vi "Get Model Info - from DLL.vi"(0 "Model Filepath":path, 4 "Models":string[](array[string]), 5 "Error (in)":errorcluster) -> (14 "DLL Inports":string[](array[string]), 15 "DLL Outports":string[](array[string]), 16 "DLL Parameters":string[](array[string]), 17 "DLL Signals":string[](array[string]), 19 "Error (out)":errorcluster)   [LabVIEW 2016, in "System Mapping Tool.lvlib"]
uses:
  System Mapping Tool.lvlib
  <vilib>/Model Interface Toolkit/Get Inport Paths.vi
  <vilib>/Model Interface Toolkit/Get Outport Paths.vi
  <vilib>/Model Interface Toolkit/Get Parameter Paths.vi
  <vilib>/Model Interface Toolkit/Get Signal Paths.vi
  <vilib>/Model Interface Toolkit/Model Interface Toolkit.lvclass
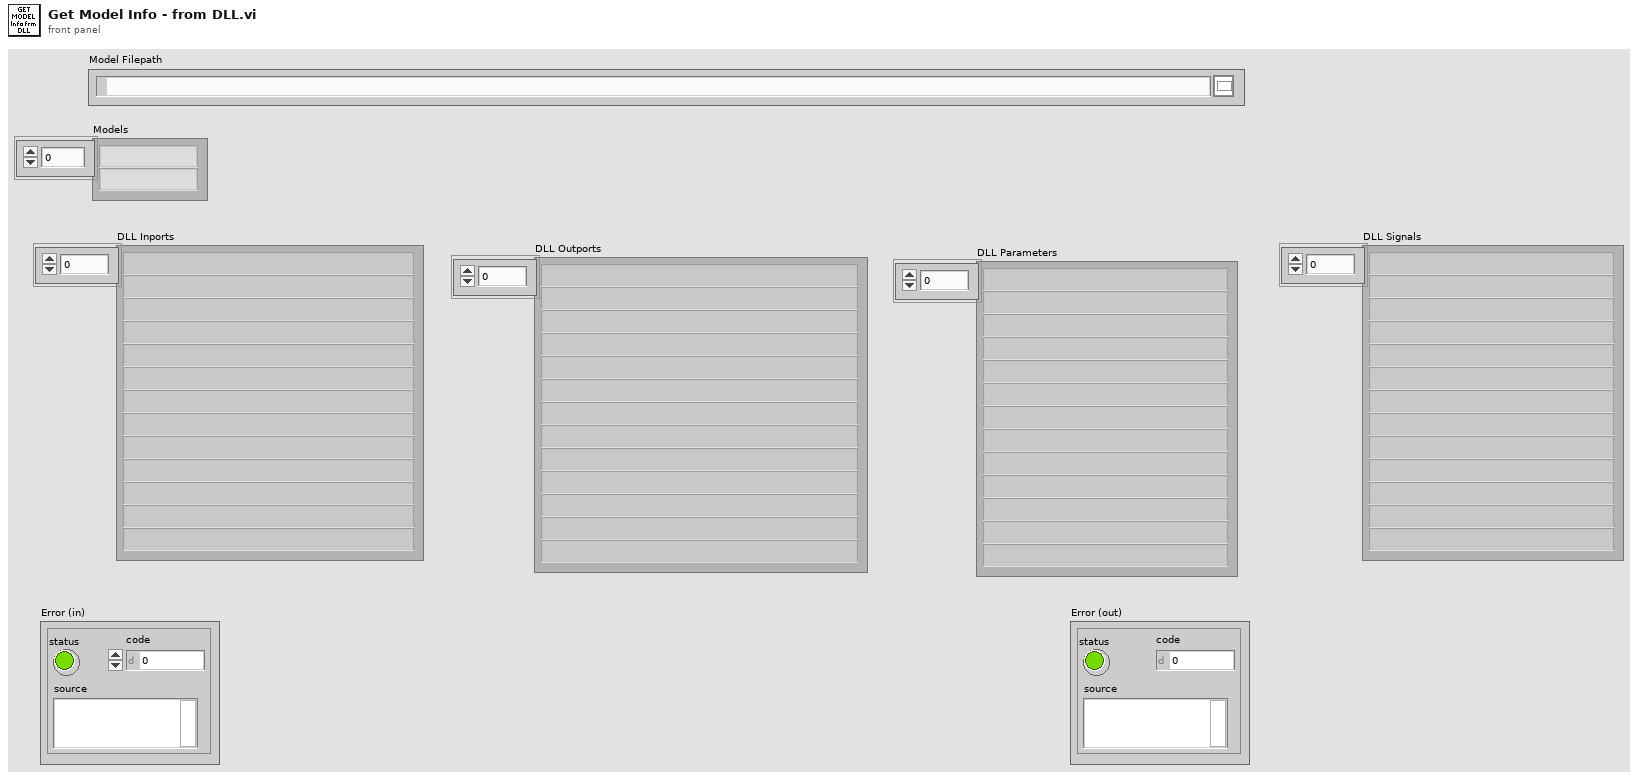
[diagram p1: front panel]
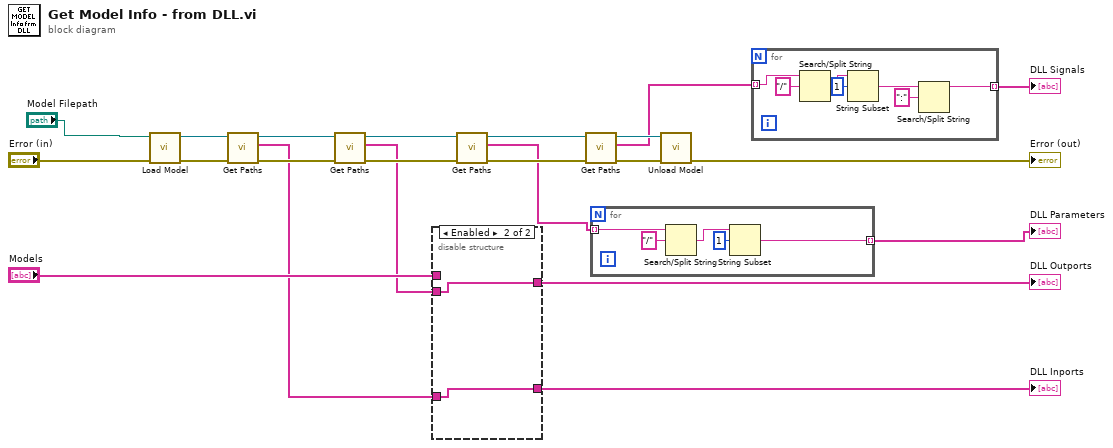
[diagram p0: block diagram]
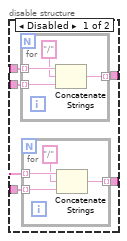
[diagram p2: hidden frame]
diagram:
  n1 = call <vilib>:"Load Model.vi"("error in (no error)"="Error (in)", "Model Path"="Model Filepath") -> ("error out"=w13:errorcluster, "Model out"=w14:refnum<class "Model Interface Toolkit.lvclass">)  [unwired: 8 in]
  n2 = call-poly <vilib>:"Get Paths.vi"("error in (no error)"=w13, "Model in"=w14) -> ("error out"=w12:errorcluster, "Inport Paths"=w9:string[], "Model out"=w15:refnum<class "Model Interface Toolkit.lvclass">)  [unwired: 7 in]
  n3 = call-poly <vilib>:"Get Paths.vi"("error in (no error)"=w12, "Model in"=w15) -> ("error out"=w11:errorcluster, "Outport Paths"=w10:string[], "Model out"=w16:refnum<class "Model Interface Toolkit.lvclass">)  [unwired: 7 in]
  n4 = disable-structure shown="Enabled" {
    disable-tunnel: w10 -> [w27 w37]
    disable-tunnel: [w26 w37] -> w20
    disable-tunnel: w9 -> [w25 w36]
    disable-tunnel: [w24 w36] -> w19
    disable-tunnel: "Models" -> [w23 _]
    frame Disabled {
      n5 = for {
        tunnel: w23 -> [w35] mode=indexing
        tunnel: w27 -> [w34] mode=indexing
        tunnel: [w32] -> w26 mode=indexing
        n6 = Concatenate Strings(w35, "/" ("string"), w34) -> (w32:string)
      }
      n7 = for {
        tunnel: w23 -> [w31] mode=indexing
        tunnel: w25 -> [w30] mode=indexing
        tunnel: [w28] -> w24 mode=indexing
        n8 = Concatenate Strings(w31, "/" ("string"), w30) -> (w28:string)
      }
    }
    frame Enabled {
    }
  }
  "DLL Inports" <- w19
  "DLL Outports" <- w20
  n9 = call-poly <vilib>:"Get Paths.vi"("error in"=w11, "Model in"=w16) -> ("error out"=w8:errorcluster, "Parameter Paths"=w4:string[], "Model out"=w6:refnum<class "Model Interface Toolkit.lvclass">)  [unwired: 7 in]
  n10 = call-poly <vilib>:"Get Paths.vi"("error in"=w8, "Model in"=w6) -> ("error out"=w7:errorcluster, "Signal Paths"=w2:string[], "Model out"=w5:refnum<class "Model Interface Toolkit.lvclass">)  [unwired: 7 in]
  n11 = for {
    tunnel: w4 -> [w42] mode=indexing
    tunnel: [w39] -> w3 mode=indexing
    n12 = Search/Split String(string=w42, search string/char (-)="/") -> (match + rest of string=w38:string)  [unwired: 1 in, 2 out]
    n13 = String Subset(string=w38, offset (0)=1) -> (substring=w39:string)  [unwired: 1 in]
  }
  "DLL Parameters" <- w3
  n14 = call <vilib>:"Unload Model.vi"("error in (no error)"=w7, "Model in"=w5) -> ("error out"=→"Error (out)":errorcluster)  [unwired: 9 in]
  n15 = for {
    tunnel: w2 -> [w47] mode=indexing
    tunnel: [w43] -> w1 mode=indexing
    n16 = Search/Split String(string=w47, search string/char (-)="/") -> (match + rest of string=w48:string)  [unwired: 1 in, 2 out]
    n17 = String Subset(string=w48, offset (0)=1) -> (substring=w45:string)  [unwired: 1 in]
    n18 = Search/Split String(string=w45, search string/char (-)=":") -> (substring before match=w43:string)  [unwired: 1 in, 2 out]
  }
  "DLL Signals" <- w1
